vi "(Sub) Power Sweep.vi"(8 "error in (no error)":errorcluster caption="에러 입력(에러 없음)", 10 "Point":dbl=10.0, 11 "Taget Voltage":dbl) -> (0 "error out":errorcluster caption="에러 출력", 2 "OFF Sweep":dbl[](array[numeric]), 3 "ON Sweep":dbl[](array[numeric]))   [LabVIEW 2017]
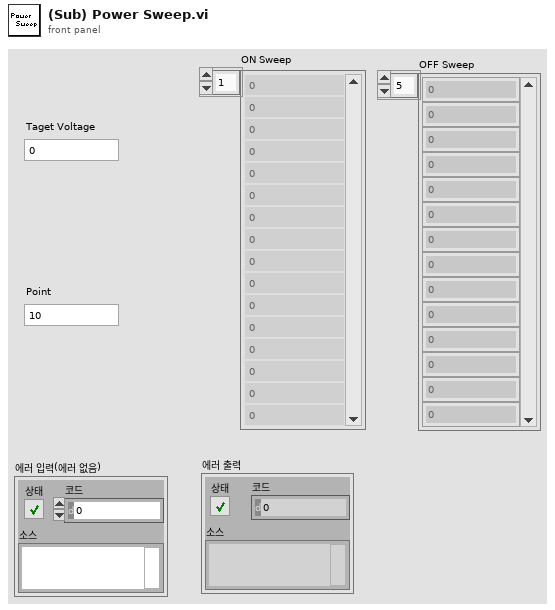
[diagram p1: front panel]
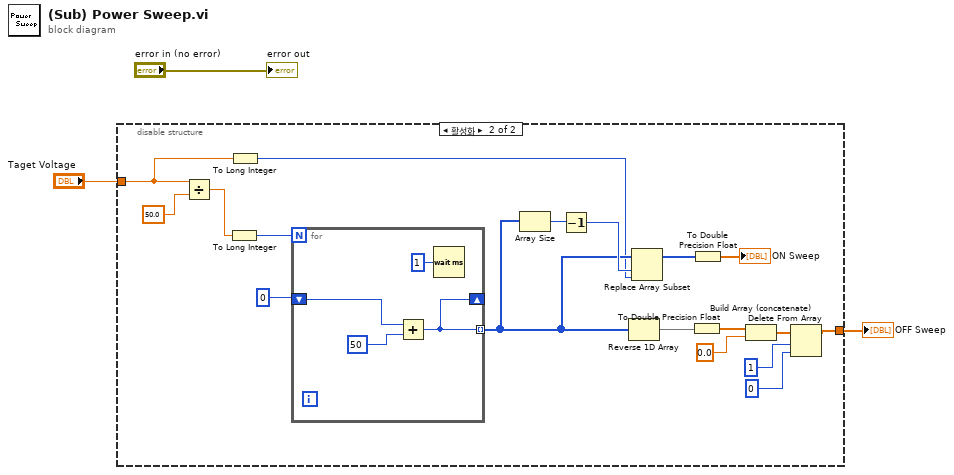
[diagram p0: block diagram]
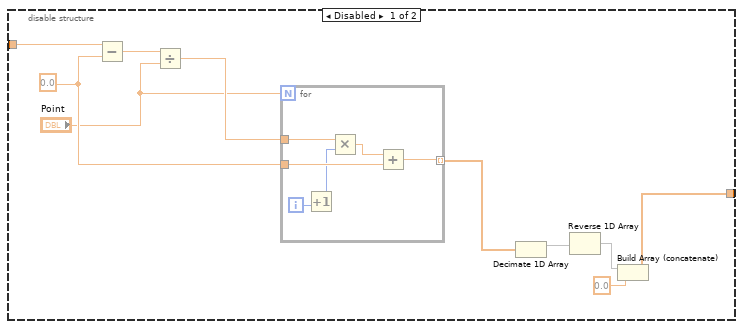
[diagram p2: hidden frame]
diagram:
  n1 = disable-structure shown="활성화" {
    disable-tunnel: "Taget Voltage" -> [w13 w23]
    disable-tunnel: [w5 w28] -> w1
    frame Disabled {
      w10 = 0.0
      n2 = Subtract(x=w13, y=w10) -> (x-y=w12:dbl)
      n3 = Divide(x=w12, y="Point") -> (x/y=w11:dbl)
      n4 = for {
        N: "Point" -> [_]
        tunnel: w11 -> [w19]
        tunnel: w10 -> [w16]
        tunnel: [w15] -> w4 mode=indexing
        i -> [w18]
        n5 = Increment(x=w18) -> (x+1=w14:i32)
        n6 = Multiply(x=w19, y=w14) -> (x*y=w17:dbl)
        n7 = Add(x=w17, y=w16) -> (x+y=w15:dbl)
      }
      n8 = Decimate 1D Array(w4) -> (w9:dbl[])  [unwired: 1 out]
      n9 = Reverse 1D Array(array=w9) -> (reversed array=w7:dbl[])
      n10 = Build Array (concatenate)(w7, 0.0) -> (w5:dbl[])
    }
    frame Enabled {
      n11 = Divide(x=w23, y=50.0) -> (x/y=w27:dbl)
      n12 = To Long Integer(number=w27) -> (32bit integer=w26:i32)
      n13 = To Long Integer(number=w23) -> (32bit integer=w22:i32)
      n14 = for {
        N: w26 -> [_]
        tunnel: [w39] -> w30 mode=indexing
        shift-right: [w39] -> _
        shift-left: 0 -> [w40]
        n15 = Add(x=w40, y=50) -> (x+y=w39:i32)
        n16 = Wait (ms)(milliseconds to wait=u32 1 ("대기 시간 (ms)")) -> ()  [unwired: 1 out]
      }
      n17 = Array Size(array=w30) -> (size(s)=w35:i32)
      n18 = Decrement(x=w35) -> (x-1=w34:i32)
      n19 = Reverse 1D Array(array=w30) -> (reversed array=w21:i32[])
      n20 = Replace Array Subset(array=w30, new element=w22, index=w34) -> (w25:i32[])
      n21 = To Double Precision Float(number=w21) -> (double precision float=w20:dbl[])
      n22 = To Double Precision Float(number=w25) -> (double precision float=→"ON Sweep":dbl[])
      n23 = Build Array (concatenate)(w20, 0.0) -> (w29:dbl[])
      n24 = Delete From Array(array=w29, length=1 ("길이"), index=0 ("인덱스")) -> (array with subset deleted=w28:dbl[])  [unwired: 1 out]
    }
  }
  "OFF Sweep" <- w1
  "error out" <- "error in (no error)"
